vi "Last Ack Creator Queue.vi"(10 "Queue":refnum<class "Queue.lvclass">, 11 "Base Queue in":refnum<class "Base Queue.lvclass">) -> (3 "Base Queue out":refnum<class "Base Queue.lvclass">)   [LabVIEW 2021, in "jettl.lvlib" / "Base Queue.lvlib" / "Base Queue.lvclass"]
uses:
  Base Queue.lvclass
  Base Queue.lvclass/Base Queue.ctl
  Queue/Queue.lvclass
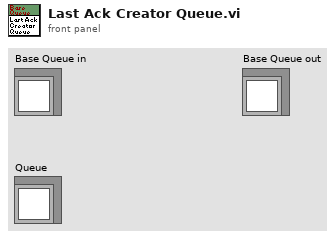
[diagram p1: front panel]
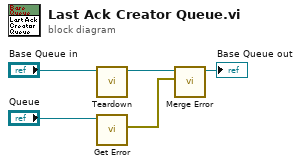
[diagram p0: block diagram]
diagram:
  n1 = call-dynamic "Teardown.vi"("Base Queue in"="Base Queue in") -> ("Base Queue out"=w1:refnum<class "Base Queue.lvclass">)  [unwired: 10 in]
  n2 = call-dynamic "Get Error.vi"("jettl in"="Queue") -> ("Error"=w3:errorcluster)  [unwired: 10 in]
  n3 = call-dynamic "Merge Error.vi"("Error"=w3, "Base Queue in"=w1) -> ("Base Queue out"=→"Base Queue out":refnum<class "Base Queue.lvclass">)  [unwired: 9 in]
